vi "设探测器列表-内容.vi"(8 "错误输出":errorcluster) -> (0 "error out":errorcluster, 2 "探测器的绑定数据":T8(array[cluster]), 3 "探测器列表内容":string[](array[string]), 5 "设备列表":T4[](array[typedef]))   [LabVIEW 2017]
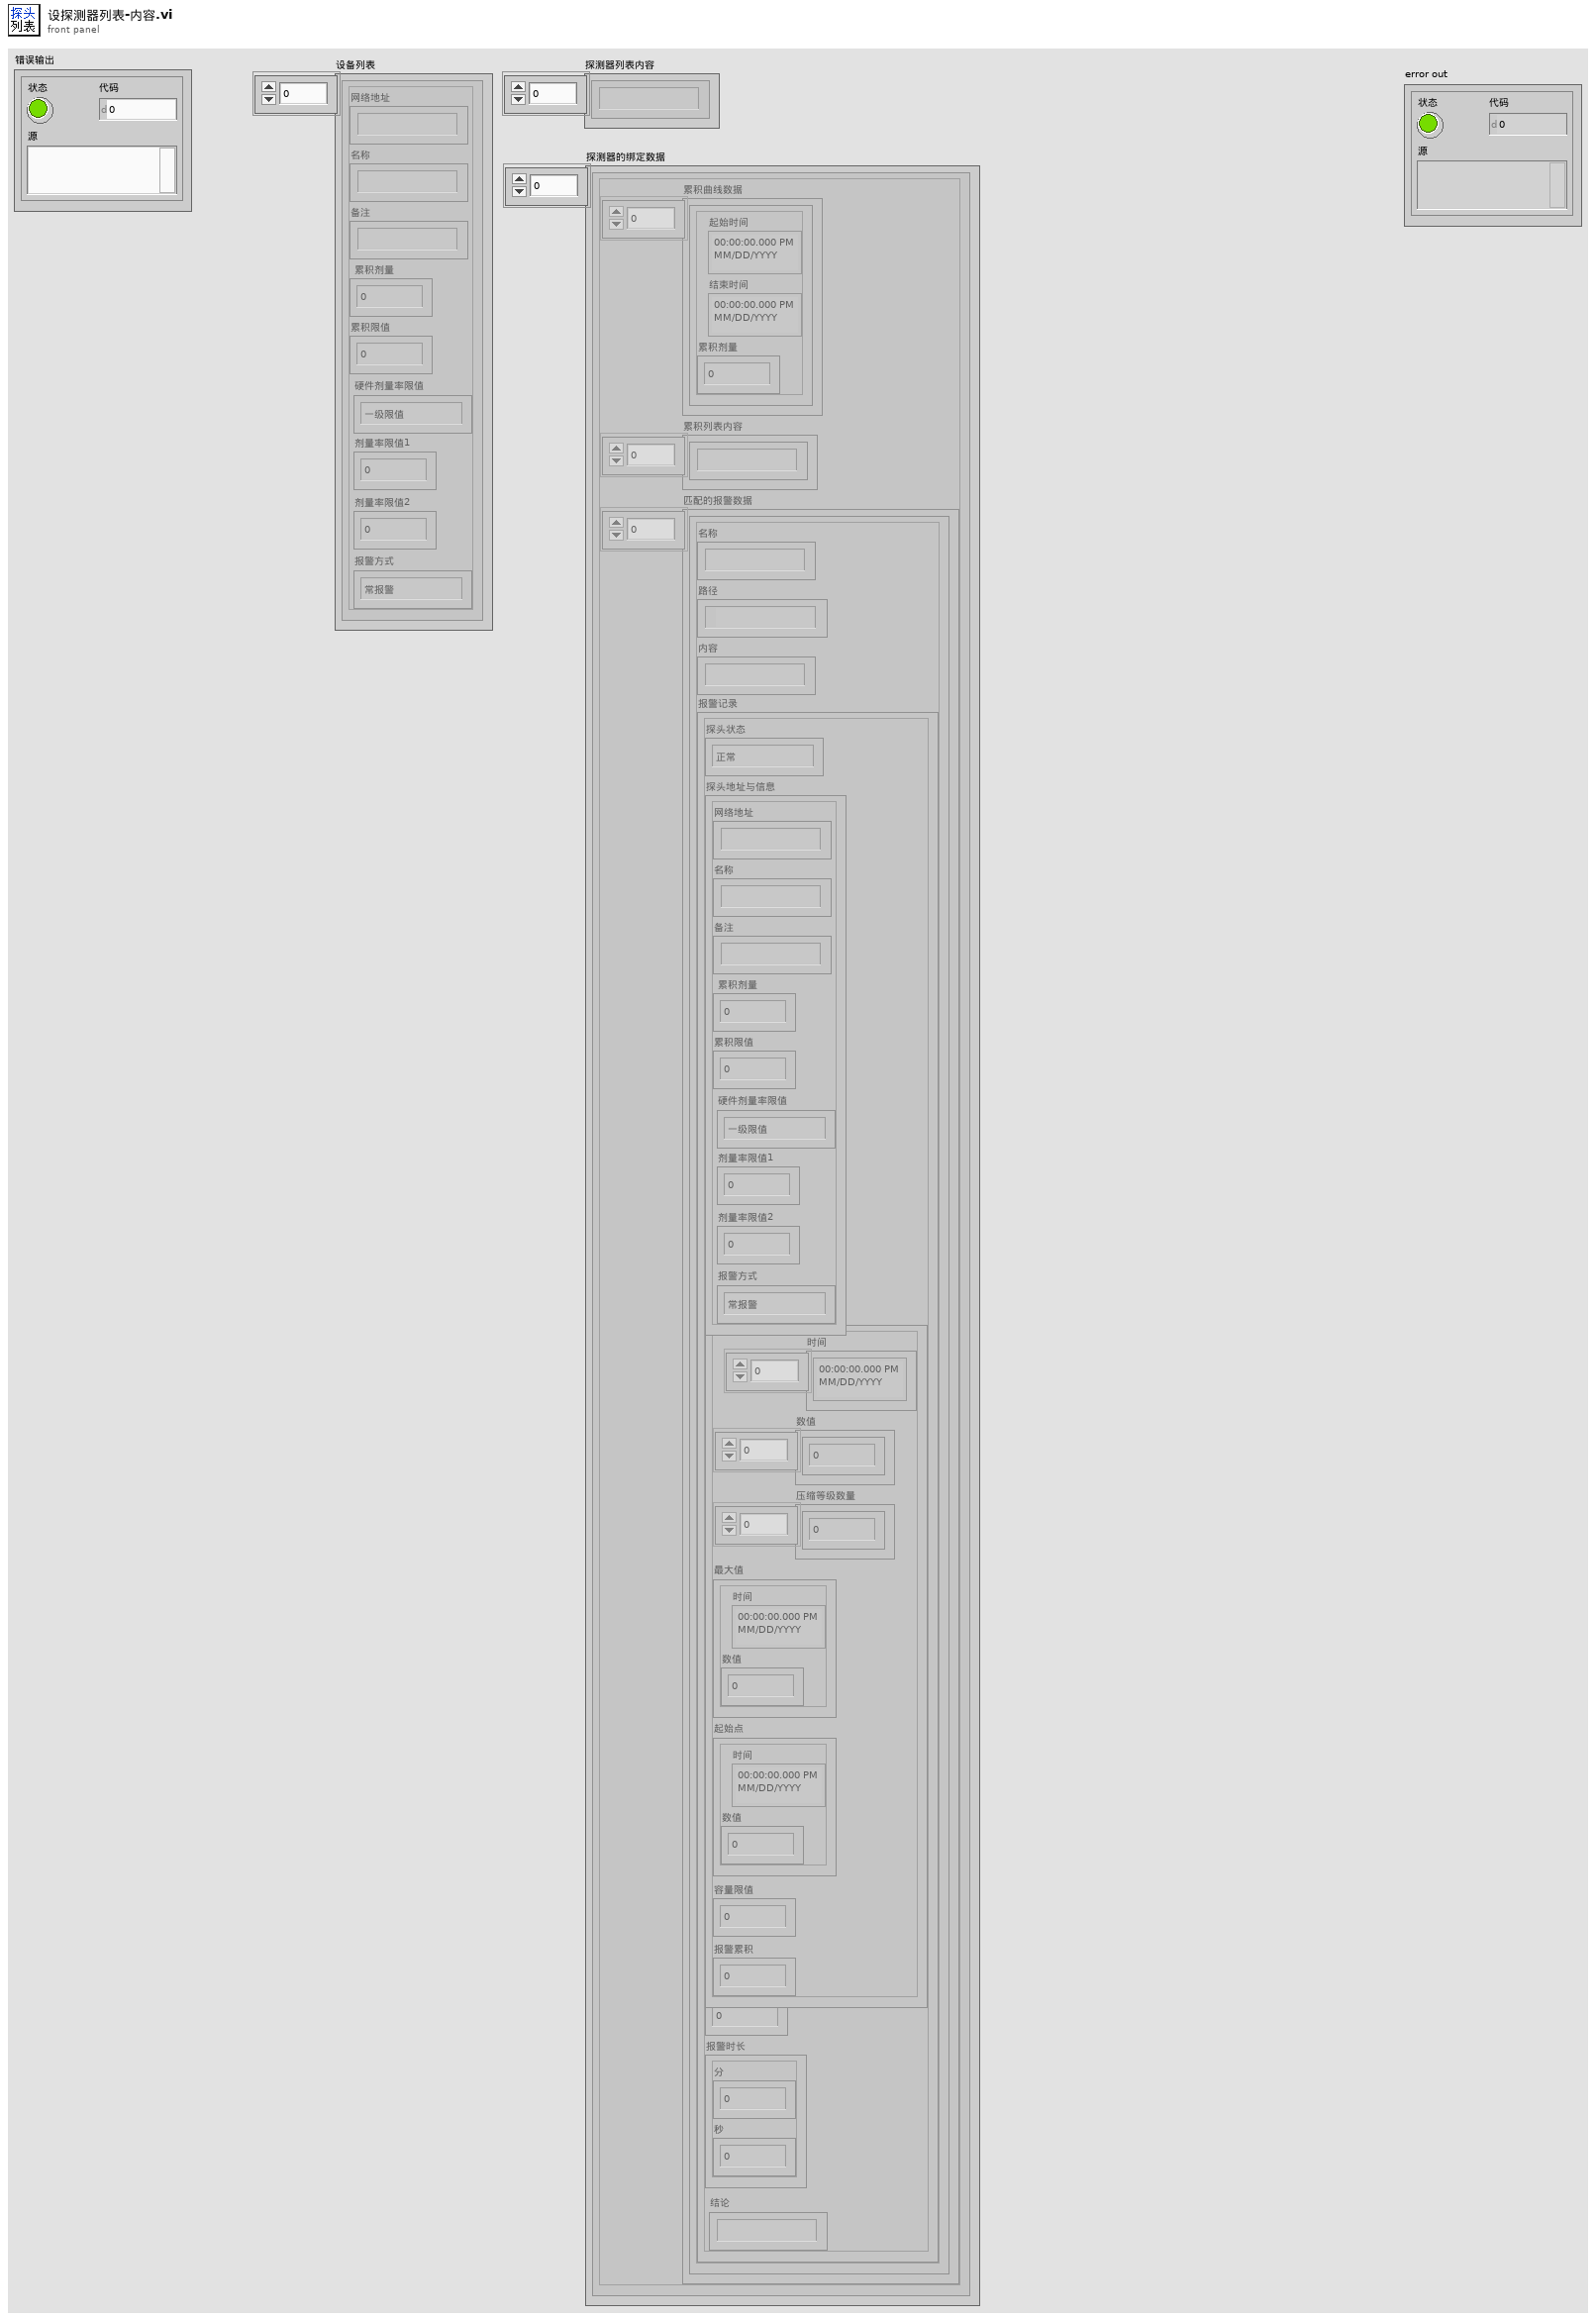
[diagram p1: front panel]
types:
  T1 = typedef "单条累积记录.ctl" = cluster{"起始时间":timestamp, "结束时间":timestamp, "累积剂量":dbl}
  T2 = typedef "通用报警记录.ctl" = cluster{"探头状态":T3, "探头地址与信息":T4, "缓存绘图数据":T7, "平均值":dbl, "报警时长":cluster{"分":u16, "秒":u16}, "结论":string}
  T3 = typedef "探头状态.ctl" = enum16{"正常", "离线", "禁用", "一级报警", "二级报警", "累积报警"}
  T4 = typedef "探测器信息.ctl" = cluster{"网络地址":string, "名称":string, "备注":string, "累积剂量":dbl, "累积限值":dbl, "硬件剂量率限值":T5, "剂量率限值1":dbl, "剂量率限值2":dbl, "报警方式":T6}
  T5 = typedef "探头剂量率限值选择.ctl" = enum16{"一级限值", "二级限值"}
  T6 = typedef "报警方式选择.ctl" = enum16{"常报警", "自动静音", "手动静音"}
  T7 = typedef "时值缓存压缩模块.lvlib/缓存数据.ctl" = cluster{"时间":timestamp[], "数值":dbl[], "压缩等级数量":i32[], "最大值":cluster{"时间":timestamp, "数值":dbl}, "起始点":cluster{"时间":timestamp, "数值":dbl}, "容量限值":i32, "报警累积":dbl}
  T8 = cluster{"累积曲线数据":T1[], "累积列表内容":string[], "匹配的报警数据":cluster{"名称":string, "路径":path, "内容":string, "报警记录":T2}[]}[]
  T9 = cluster{"名称":string, "路径":path, "内容":string, "报警记录":T2}
  T10 = typedef "DB动作类型.ctl" = enum16{"DB-文件初始化+连接", "DB-断开连接", "DB-结构初始化", "DB-加载设备", "DB-检查连接状态", "设备-登记新设备+数据表", "设备-删除设备", "设备-修改网址", "设备-修改名称+转移数据", "设备-修改备注", "设备-修改限值", "设备-累积校准", "设备-重排", "数据-获取全部", "数据-删除数据", "数据-写改累积记录+改累积剂量", "读变量-全部设备"}
  T11 = typedef "DB动作与数据.ctl" = cluster{"动作类型":T10, "输入数据":variant}
  T12 = cluster{"名称":string, "路径":path, "内容":string, "报警记录":T2}[]
  T13 = enum16{"绝对差值", "取整+1s", "取整+1m", "取整+1h", "取整+1d"}
  T14 = cluster{"累积记录数据":T1[], string[], cluster{"名称":string, "路径":path, "内容":string, "报警记录":T2}[]}
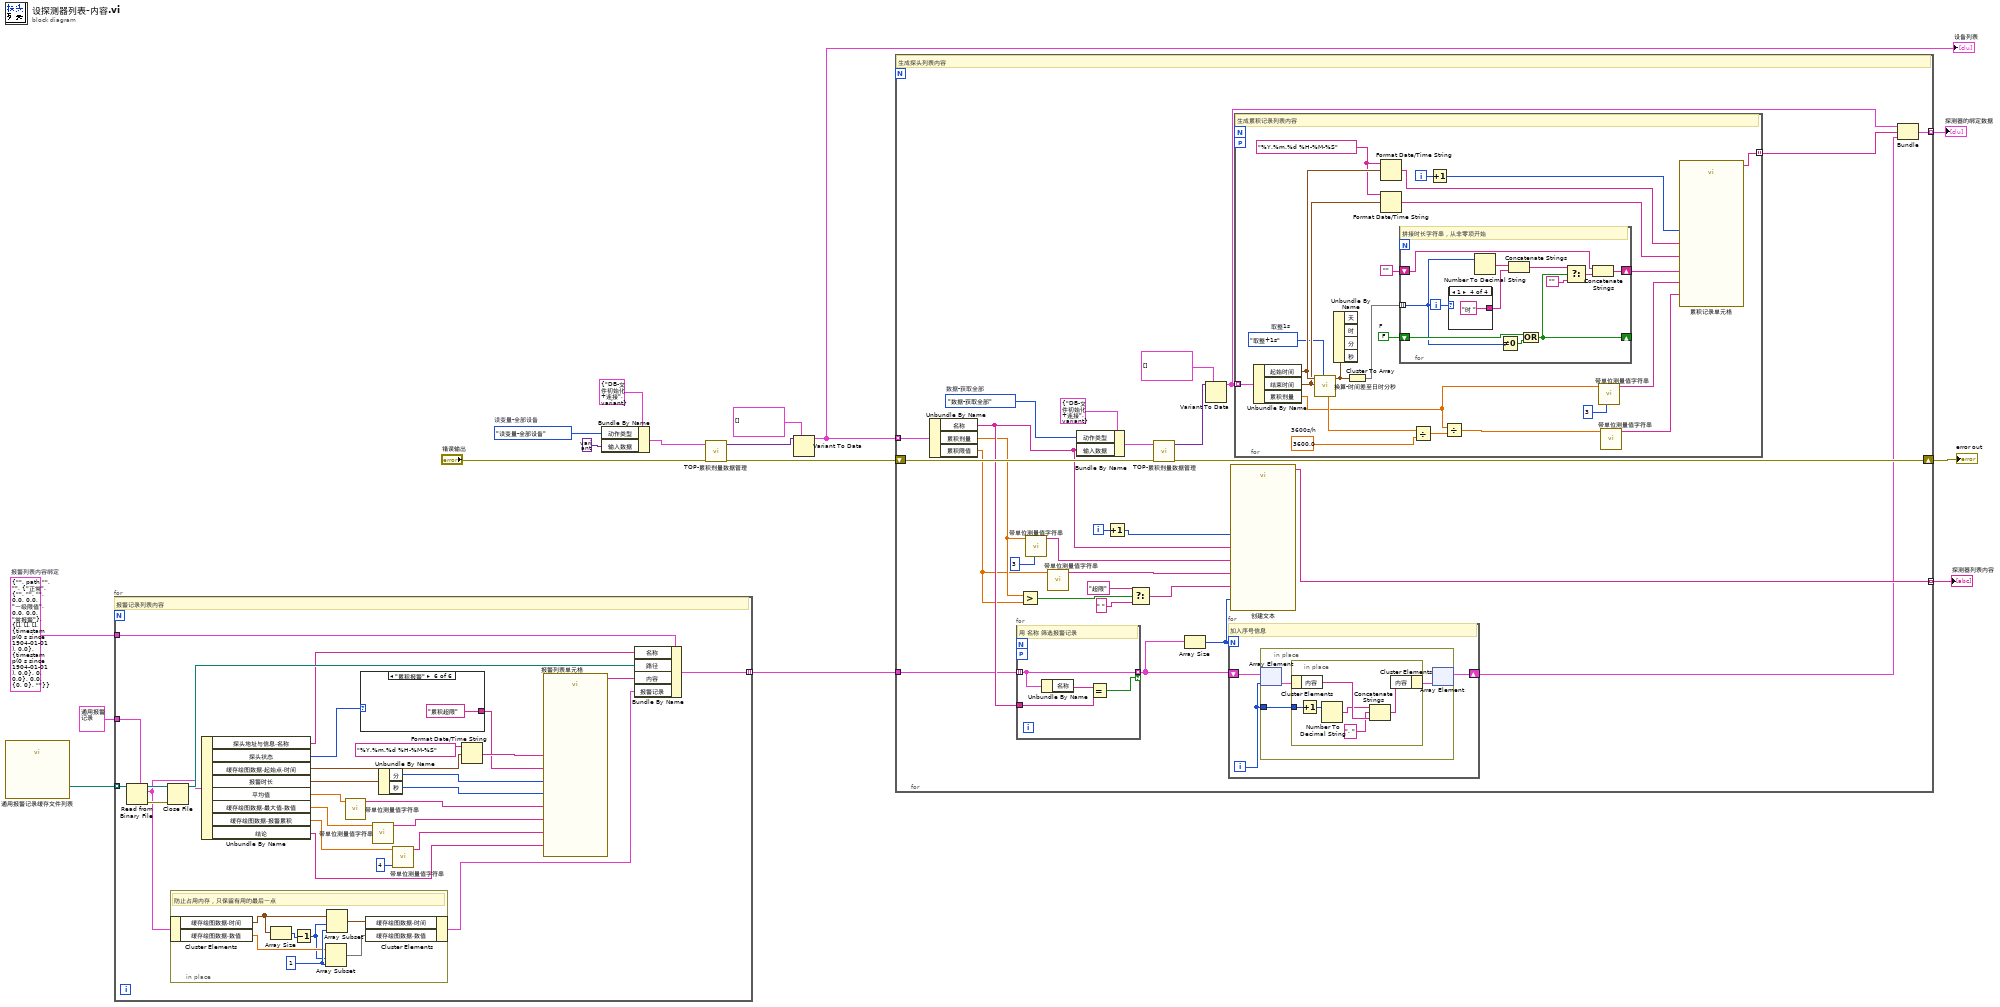
[diagram p0: block diagram]
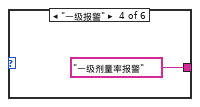
[diagram p5: hidden frame]
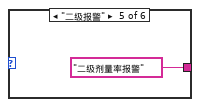
[diagram p6: hidden frame]
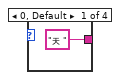
[diagram p7: hidden frame]
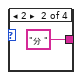
[diagram p8: hidden frame]
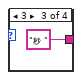
[diagram p9: hidden frame]
diagram:
  w3 = T9 {"名称"="", "路径"=path "", "内容"="", "报警记录"={"探头状态"=enum."正常", "探头地址与信息"={"网络地址"="", "名称"="", "备注"="", "累积剂量"=0.0, "累积限值"=0.0, "硬件剂量率限值"=enum."一级限值", "剂量率限值1"=0.0, "剂量率限值2"=0.0, "报警方式"=enum."常报警"}, "缓存绘图数据"={"时间"=[], "数值"=[], "压缩等级数量"=[], "最大值"={"时间"=timestamp(0 s since 1904-01-01), "数值"=0.0}, "起始点"={"时间"=timestamp(0 s since 1904-01-01), "数值"=0.0}, "容量限值"=0, "报警累积"=0.0}, "平均值"=0.0, "报警时长"={"分"=0, "秒"=0}, "结论"=""}}  # 报警列表内容绑定
  w14 = DB动作类型."读变量-全部设备"  # 读变量-全部设备
  n1 = call "通用报警记录缓存文件列表.vi"() -> ("报警记录文件"=w5:path[])  [unwired: 11 in]
  n2 = for {
    tunnel: w5 -> [w43] mode=indexing
    tunnel: T2 {"探头状态"=enum."正常", "探头地址与信息"={"网络地址"="", "名称"="", "备注"="", "累积剂量"=0.0, "累积限值"=0.0, "硬件剂量率限值"=enum."一级限值", "剂量率限值1"=0.0, "剂量率限值2"=0.0, "报警方式"=enum."常报警"}, "缓存绘图数据"={"时间"=[], "数值"=[], "压缩等级数量"=[], "最大值"={"时间"=timestamp(0 s since 1904-01-01), "数值"=0.0}, "起始点"={"时间"=timestamp(0 s since 1904-01-01), "数值"=0.0}, "容量限值"=0, "报警累积"=0.0}, "平均值"=0.0, "报警时长"={"分"=0, "秒"=0}, "结论"=""} ("报警记录") -> [w42]
    tunnel: w3 -> [w33]
    tunnel: [w30] -> w1 mode=indexing
    # "报警记录列表内容"
    n3 = Read from Binary File(5:w42, 11:w43) -> (0:w40:errorcluster, 2:w29:T2, 3:w41:refnum<file>)  [unwired: 4 in, 1 out]
    n4 = Close File(refnum=w41, error in=w40) -> (path=w32:path)  [unwired: 1 out]
    n5 = in-place {
      w50 = 1 ("长度")
      # "防止占用内存，只保留有用的最后一点"
      n6 = in-place-cluster #1(w29) -> ("缓存绘图数据.时间"=w46:timestamp[], "缓存绘图数据.数值"=w47:dbl[])
      n7 = Array Size(array=w46) -> (size(s)=w45:i32)
      n8 = Decrement(x=w45) -> (x-1=w44:i32)
      n9 = Array Subset(array=w47, index=w44, length=w50) -> (w48:dbl[])
      n10 = Array Subset(array=w46, index=w44, length=w50) -> (w49:timestamp[])
      n11 = in-place-cluster #1("缓存绘图数据.时间"=w49, "缓存绘图数据.数值"=w48) -> (w28:T2)
    }
    n12 = Unbundle By Name(w29) -> ("探头地址与信息.名称"=w26:string, "探头状态"=w39:T3, "缓存绘图数据.起始点.时间"=w37:timestamp, "报警时长"=w36:cluster{"分":u16, "秒":u16}, "平均值"=w35:dbl, "缓存绘图数据.最大值.数值"=w34:dbl, "缓存绘图数据.报警累积"=w27:dbl, "结论"=w18:string)
    n13 = call "带单位测量值字符串.vi"("测量值"=w35) -> ("结果"=w21:string)  [unwired: 10 in]
    n14 = case shown="\"累积报警\"" w39 {
      tunnel: [_ _ _ "一级剂量率报警" "二级剂量率报警" "累积超限"] -> w24
      frame "正常", Default {
      }
      frame "离线" {
      }
      frame "禁用" {
      }
      frame "一级报警" {
      }
      frame "二级报警" {
      }
      frame "累积报警" {
      }
    }
    n15 = call "带单位测量值字符串.vi"("测量值"=w34) -> ("结果"=w20:string)  [unwired: 10 in]
    n16 = Unbundle By Name(w36) -> ("分"=w23:u16, "秒"=w22:u16)
    n17 = call "带单位测量值字符串.vi"("精度(2)"=i16 4, "测量值"=w27) -> ("结果"=w19:string)  [unwired: 9 in]
    n18 = Format Date/Time String(time format string (%c)="%Y.%m.%d %H-%M-%S" ("时间格式字符串(%c)"), seconds (now)=w37) -> (date/time string=w25:string)  [unwired: 1 in]
    n19 = call "报警列表单元格"("秒"=w22, "最大值"=w20, "结论"=w18, "起始时间"=w25, "类型"=w24, "分"=w23, "平均值"=w21, "报警累积"=w19) -> ("Result"=w31:string)  [unwired: 6 in, 1 out]
    n20 = Bundle By Name(cluster=w33, "名称"=w26, "路径"=w32, "内容"=w31, "报警记录"=w28) -> (w30:T9)
  }
  n21 = Bundle By Name(cluster=T11 {"动作类型"=enum."DB-文件初始化+连接", "输入数据"=variant} ("DB动作集"), "动作类型"=w14, "输入数据"=variant) -> (w15:T11)
  n22 = call "TOP-累积剂量数据管理.vi"("错误输出"="错误输出", "DB动作集"=w15) -> ("error out"=w8:errorcluster, "输出数据"=w12:variant)  [unwired: 8 in]
  n23 = Variant To Data(type=T4[] [] ("探测器清单"), Variant=w12) -> (data=w10:T4[])  [unwired: 1 in, 1 out]
  "设备列表" <- w10
  n24 = for {
    tunnel: w10 -> [w67] mode=indexing
    tunnel: [w79] -> w6 mode=indexing
    shift-right: [w77] -> w7
    shift-left: w8 -> [w78]
    tunnel: w1 -> [w65]
    tunnel: [w62] -> w2 mode=indexing
    i -> [w81]
    w74 = DB动作类型."数据-获取全部"  # 数据-获取全部
    # "生成探头列表内容"
    n25 = Unbundle By Name(w67) -> ("名称"=w66:string, "累积剂量"=w60:dbl, "累积限值"=w59:dbl)
    n26 = for {
      tunnel: w66 -> [w96]
      tunnel: w65 -> [w95] mode=indexing
      tunnel: [w95] -> w64 mode=indexing if=w94
      workers-P: _ -> [_]
      # "用 名称 筛选报警记录"
      n27 = Unbundle By Name(w95) -> ("名称"=w97:string)
      n28 = Equal?(x=w97, y=w96) -> (x = y?=w94:bool)
    }
    n29 = Greater?(x=w60, y=w59) -> (0:w58:bool)
    n30 = call "带单位测量值字符串.vi"("精度(2)"=i16 3, "测量值"=w60) -> ("结果"=w71:string)  [unwired: 9 in]
    n31 = call "带单位测量值字符串.vi"("测量值"=w59) -> ("结果"=w70:string)  [unwired: 10 in]
    n32 = Bundle By Name(cluster=T11 {"动作类型"=enum."DB-文件初始化+连接", "输入数据"=variant} ("DB动作集"), "动作类型"=w74, "输入数据"=w66) -> (w73:T11)
    n33 = Increment(x=w81) -> (x+1=w80:i32)
    n34 = Select(t="超限" ("字符串"), s=w58, f=" " ("字符串")) -> (s? t:f=w55:string)
    n35 = call "TOP-累积剂量数据管理.vi"("错误输出"=w78, "DB动作集"=w73) -> ("error out"=w77:errorcluster, "输出数据"=w76:variant)  [unwired: 8 in]
    n36 = Array Size(array=w64) -> (size(s)=w61:i32)
    n37 = Variant To Data(type=T1[] [] ("累积记录数据"), Variant=w76) -> (data=w68:T1[])  [unwired: 1 in, 1 out]
    n38 = for {
      N: w61 -> [_]
      shift-right: [w82] -> w63
      shift-left: w64 -> [w84]
      i -> [w83]
      # "加入序号信息"
      n39 = in-place {
        in-place-border: w83 -> [w86]
        n40 = in-place-array #2(w84, w83) -> (w87:T9)
        n41 = in-place {
          in-place-border: w86 -> [w92]
          n42 = in-place-cluster #3(w87) -> ("内容"=w93:string)
          n43 = Increment(x=w92) -> (x+1=w91:i32)
          n44 = Number To Decimal String(number=w91) -> (decimal integer string=w90:string)  [unwired: 1 in]
          n45 = Concatenate Strings(w90, ". " ("字符串"), w93) -> (w88:string)
          n46 = in-place-cluster #3("内容"=w88) -> (w85:T9)
        }
        n47 = in-place-array #2(w85) -> (w82:T12)  [unwired: 1 out]
      }
    }
    n48 = call "创建文本"("累积限值Sv"=w70, "报警记录条数"=w61, "序号"=w80, "名称"=w66, "累积剂量Sv"=w71, "超限提示"=w55) -> ("Result"=w79:string)  [unwired: 8 in, 1 out]
    n49 = for {
      tunnel: w68 -> [w120] mode=indexing
      workers-P: _ -> [_]
      tunnel: [w104] -> w69 mode=indexing
      i -> [w111]
      w98 = T13."取整+1s"  # 取整1s
      w103 = FALSE  # F
      w112 = "%Y.%m.%d %H-%M-%S" ("时间格式字符串(%c)")
      w118 = 3600.0  # 3600s/h
      # "生成累积记录列表内容"
      n50 = Unbundle By Name(w120) -> ("起始时间"=w114:timestamp, "结束时间"=w113:timestamp, "累积剂量"=w115:dbl)
      n51 = call "换算-时间差至日时分秒.vi"("时长模式"=w98, "时间1"=w113, "时间2"=w114) -> ("时长"=w105:cluster{"天":i32, "时":i32, "分":i32, "秒":i32}, "时长 s"=w119:dbl)  [unwired: 7 in]
      n52 = Unbundle By Name(w105) -> ()  [unwired: 4 out]
      n53 = Cluster To Array(cluster=w105) -> (array=w101:i32[])
      n54 = Format Date/Time String(time format string (%c)=w112, seconds (now)=w114) -> (date/time string=w109:string)  [unwired: 1 in]
      n55 = Format Date/Time String(time format string (%c)=w112, seconds (now)=w113) -> (date/time string=w108:string)  [unwired: 1 in]
      n56 = for {
        shift-right: [w128] -> w100
        shift-left: "" -> [w129]
        shift-right: [w122] -> _
        shift-left: w103 -> [w127]
        tunnel: w101 -> [w121] mode=indexing
        i -> [w132]
        # "拼接时长字符串，从非零项开始"
        n57 = case shown="1" w132 {
          tunnel: ["天 " "分 " "秒 " "时 "] -> w131
          frame 0, Default {
          }
          frame 2 {
          }
          frame 3 {
          }
          frame 1 {
          }
        }
        n58 = Number To Decimal String(number=w121) -> (decimal integer string=w130:string)  [unwired: 1 in]
        n59 = Not Equal To 0?(x=w121) -> (x != 0?=w126:bool)
        n60 = Concatenate Strings(w130, w131) -> (w125:string)
        n61 = Or(x=w127, y=w126) -> (x .or. y?=w122:bool)
        n62 = Select(t=w125, s=w122, f="") -> (s? t:f=w123:string)
        n63 = Concatenate Strings(w129, w123) -> (w128:string)
      }
      n64 = Divide(x=w119, y=w118) -> (x/y=w117:dbl)
      n65 = Increment(x=w111) -> (x+1=w110:i32)
      n66 = Divide(x=w115, y=w117) -> (x/y=w116:dbl)
      n67 = call "带单位测量值字符串.vi"("精度(2)"=i16 3, "测量值"=w115) -> ("结果"=w107:string)  [unwired: 9 in]
      n68 = call "带单位测量值字符串.vi"("测量值"=w116) -> ("结果"=w106:string)  [unwired: 10 in]
      n69 = call "累积记录单元格"("时长"=w100, "平均Sv/h"=w106, "序号"=w110, "起始时间"=w109, "结束时间"=w108, "累积Sv"=w107) -> ("Result"=w104:string)  [unwired: 8 in, 1 out]
    }
    n70 = Bundle("累积记录数据"=w68, w69, w63) -> (w62:T14)  [unwired: 1 in]
  }
  "error out" <- w7
  "探测器列表内容" <- w6
  "探测器的绑定数据" <- w2
